vi "Main_24a.vi"() -> ()   [LabVIEW 2023]
uses:
  RB ENUM_Position ID.ctl
  Cluster _Point Location.ctl
  0c90424e-a446-4045-a5ae-fd3bd7481f50.vi
  <vilib>/Comparison/Equal/Equal Functor/Equal Functor.lvclass
panel:
  in  "Description":string="--- Day 24: Blizzard Basin ---\nWith everything replanted for next year (and with elephants and monkeys to tend the grove), you and the Elves leave for the extraction point.\n\nPartway up the mountain that shields the grove is a flat, open area that serves as the extraction point. It's a bit of a climb, but nothing the expedition can't handle.\n\nAt least, that would normally be true; now that the mountain is covered in snow, things have become more difficult than the Elves are used to.\n\nAs the expedition reaches a valley that must be traversed to reach the extraction site, you find that strong, turbulent winds are pushing small blizzards of snow and sharp ice around the valley. It's a good thing everyone packed warm clothes! To make it across safely, you'll need to find a way to avoid them.\n\nFortunately, it's easy to see all of this from the entrance to the valley, so you make a map of the valley and the blizzards (your puzzle input). For example:\n\n#.#####\n#.....#\n#>....#\n#.....#\n#...v.#\n#.....#\n#####.#\nThe walls of the valley are drawn as #; everything else is ground. Clear ground - where there is currently no blizzard - is drawn as .. Otherwise, blizzards are drawn with an arrow indicating their direction of motion: up (^), down (v), left (<), or right (>).\n\nThe above map includes two blizzards, one moving right (>) and one moving down (v). In one minute, each blizzard moves one position in the direction it is pointing:\n\n#.#####\n#.....#\n#.>...#\n#.....#\n#.....#\n#...v.#\n#####.#\nDue to conservation of blizzard energy, as a blizzard reaches the wall of the valley, a new blizzard forms on the opposite side of the valley moving in the same direction. After another minute, the bottom downward-moving blizzard has been replaced with a new downward-moving blizzard at the top of the valley instead:\n\n#.#####\n#...v.#\n#..>..#\n#.....#\n#.....#\n#.....#\n#####.#\nBecause blizzards are made of tiny snowflakes, they pass right through each other. After another minute, both blizzards temporarily occupy the same position, marked 2:\n\n#.#####\n#.....#\n#...2.#\n#.....#\n#.....#\n#.....#\n#####.#\nAfter another minute, the situation resolves itself, giving each blizzard back its personal space:\n\n#.#####\n#.....#\n#....>#\n#...v.#\n#.....#\n#.....#\n#####.#\nFinally, after yet another minute, the rightward-facing blizzard on the right is replaced with a new one on the left facing the same direction:\n\n#.#####\n#.....#\n#>....#\n#.....#\n#...v.#\n#.....#\n#####.#\nThis process repeats at least as long as you are observing it, but probably forever.\n\nHere is a more complex example:\n\n#.######\n#>>.<^<#\n#.<..<<#\n#>v.><>#\n#<^v^^>#\n######.#\nYour expedition begins in the only non-wall position in the top row and needs to reach the only non-wall position in the bottom row. On each minute, you can move up, down, left, or right, or you can wait in place. You and the blizzards act simultaneously, and you cannot share a position with a blizzard.\n\nIn the above example, the fastest way to reach your goal requires 18 steps. Drawing the position of the expedition as E, one way to achieve this is:\n\nInitial state:\n#E######\n#>>.<^<#\n#.<..<<#\n#>v.><>#\n#<^v^^>#\n######.#\n\nMinute 1, move down:\n#.######\n#E>3.<.#\n#<..<<.#\n#>2.22.#\n#>v..^<#\n######.#\n\nMinute 2, move down:\n#.######\n#.2>2..#\n#E^22^<#\n#.>2.^>#\n#.>..<.#\n######.#\n\nMinute 3, wait:\n#.######\n#<^<22.#\n#E2<.2.#\n#><2>..#\n#..><..#\n######.#\n\nMinute 4, move up:\n#.######\n#E<..22#\n#<<.<..#\n#<2.>>.#\n#.^22^.#\n######.#\n\nMinute 5, move right:\n#.######\n#2Ev.<>#\n#<.<..<#\n#.^>^22#\n#.2..2.#\n######.#\n\nMinute 6, move right:\n#.######\n#>2E<.<#\n#.2v^2<#\n#>..>2>#\n#<....>#\n######.#\n\nMinute 7, move down:\n#.######\n#.22^2.#\n#<vE<2.#\n#>>v<>.#\n#>....<#\n######.#\n\nMinute 8, move left:\n#.######\n#.<>2^.#\n#.E<<.<#\n#.22..>#\n#.2v^2.#\n######.#\n\nMinute 9, move up:\n#.######\n#<E2>>.#\n#.<<.<.#\n#>2>2^.#\n#.v><^.#\n######.#\n\nMinute 10, move right:\n#.######\n#.2E.>2#\n#<2v2^.#\n#<>.>2.#\n#..<>..#\n######.#\n\nMinute 11, wait:\n#.######\n#2^E^2>#\n#<v<.^<#\n#..2.>2#\n#.<..>.#\n######.#\n\nMinute 12, move down:\n#.######\n#>>.<^<#\n#.<E.<<#\n#>v.><>#\n#<^v^^>#\n######.#\n\nMinute 13, move down:\n#.######\n#.>3.<.#\n#<..<<.#\n#>2E22.#\n#>v..^<#\n######.#\n\nMinute 14, move right:\n#.######\n#.2>2..#\n#.^22^<#\n#.>2E^>#\n#.>..<.#\n######.#\n\nMinute 15, move right:\n#.######\n#<^<22.#\n#.2<.2.#\n#><2>E.#\n#..><..#\n######.#\n\nMinute 16, move right:\n#.######\n#.<..22#\n#<<.<..#\n#<2.>>E#\n#.^22^.#\n######.#\n\nMinute 17, move down:\n#.######\n#2.v.<>#\n#<.<..<#\n#.^>^22#\n#.2..2E#\n######.#\n\nMinute 18, move down:\n#.######\n#>2.<.<#\n#.2v^2<#\n#>..>2>#\n#<....>#\n######E#\nWhat is the fewest number of minutes required to avoid the blizzards and reach the goal?"
  out "Array":T1[][](array[typedef])
  in  "Example 2":string="#.######\n#>>.<^<#\n#.<..<<#\n#>v.><>#\n#<^v^^>#\n######.#"
  out "Answer":i32
  in  "Puzzle":string="#.######################################################################################################################################################\n#>v<<.^vvv^vv.^^>>v<>><v^<<.>^>v>v<v^vvvvvv^><^<vv<^^^v<vv>vvv.^v>.<>>v^v><<>^<<^vv<<>><<v<v<^v<..^>>vv^><<<v<^^><<<>>>vvv^.^.v>.^v^^.vv>^vv^>^^^><v<<<#\n#.<<v^><<.<>>>>^.<^<^^<>>^.^^.^v<vvv>>vv<^>.>>^^<<<^^>><^><<<v^>v.^^<.<<^v^>^^>.^.v^>.><<vv^>><>^....^<vv^><<^>v<v<^vvv<v<<><^vv<^>v^^^^^^^.^vv<^^<vvv<#\n#<>.v^.v<^><><v^^>>^><.v>^v^vv><><>>^>^v<^>>v^>^vvv^v..>vv>.^vv^<^.<.<v>>^<><v>^>^v..^>^><>vvv<v>^.>>^^<v^v>^<^vv.>.^v><v>v^>.^v<v>.<<vvv><^v^<^<^<vv<>#\n#>v..v^<^^v<><^^>vv>v^^^<^.^<<><^^^v>^<^v<<^>^<<.^><<^>>v^.v.><>>^<<><^^>>v>.^<^<vv><<>..>>v^^^>v>^<vv>.^>^<.^^v<>v>^.^>^^>.^v^>>^v>>>^<<^.^>><>v^>v>v.#\n#>^^^^^v^>>>^^v^v^v>v^v<v^.><<.^..v<^<^<^><<><<<>>v<<>><<^v^^>v>v<>.<vv>^<<<><.v<v<>>v^v<>>^v><.v>><<v><v<vv<<^^<><.^>v>^<^<^>^^.<.v>v^>>>><<<^v.vv<.<>#\n#>vv<vv^v<.<<v><<<^v>v<><vv<<vv<<.^.v>>v>.>v<^<<>v>>vv>..>v<^.v<.^<.>.<<<>>>^v>.^>>>>><<<^>..>>>^<^<>^>><>^><><v>v<<<v^.vvvv<v>>vv^>>>^.v^<>^><.<v>>v>>#\n#>>v.>><v^>v^v.<^.<vvv<<<v<>.^^v<<^^>>^^v^^.^.<>^vv^>>v<>^>v^.vv^v>.v^<>>v<<v<^>^vv^^v^><>v>.^<v<v<.^>>vvv>v^<^vv^<v^<<>^<v<>v<<v<<>v^v><>^vv^<<<^v>^>>#\n#<^<^>><<.<<.><<v>vv>v^v<<>..v<^>v^<.vv><v^<<<.v>v>>><<^.<v^vvv^<^v<<^^^^<v<<.<<^><v.<>>^><v>..<><vvv<.<>><.v>.v><<>vv<>.<<v.>><>>v<v^>^>>..>.<<^>^>^.>#\n#<v.>v>v<>>v^v>^v<^vv>^^>^vv>v<^^vv><^.<v<^<v>^>^v<v.<^<>^>>>vvvv<v>>^^<v.^v<^^<.<<<><v^<>^^<vvv><<>...^<><>^>vvv^^v..v..v^><^<>^>vv><v<^^vv^vvv>v^<v><#\n#<^^^^.>v>><<>v<vv<^<<^>v..vv^vvv>>>v<<^vv^^><^>^>^v.<<^v^^><vv>.>v..v.^v><^<^>>^>vv<<v.v>.<.>^.>>>^>>^^v^>^<.<><v>v^.^..<>.>^<^^<v.^v>^^^<<^v>>.>vv<v>#\n#>^^v>v.<v<<v..>><>..^v><>.^<v.>vv<>v^^>v.^v<<<vv>>v.^>><<^<v><v^.>>>^v>^>>v<<...<^^^vv.v^><<<>^^v<v^>v<v>.vv^vv.>>v<>><>v><vv>^>>v^..vv>v>^^>vvv>.>^v<#\n#<v>^^.<.^vv^<>^vv<<<<<vv^<^^<>v>^vv<>v<<>vv^<<v><<.^^..>.^>vv<^<>>^.<<<<<>.v>v><>.>v>v^<>^>vvv>.<^v^.>^<<v<^vvv^>v><<v^>.^><^><>v.^^<><vv<>.v..^<<v^>>#\n#<>^.>.><><v^<v>v>^<<>^v..<.<><>>^.vv>v.vv.>><>v^>.^><.<v.>v..^^v.^v^>^<^^<>>>v<^>>v<^<v^^^v<^v.vv<v^.><^^v^>^^^<.>.<v<.<v>^.><^^<v^<<^^v<.>>v>.vvv>v>>#\n#<v><v.^^<>v>.>^^^^>v<<v..v>><>v^.>^^<^>v<>v^v<v^<><^<>v>v^.<.^v^<^<>v^^<<^v><^.>^.v><><>>^v^v><.>v><<>v>v^.vvv><>^>>v^<<^v>^vv><><.^^>>vv^^v><^..>^v<>#\n#>v><^<vv^v>v><>v^<<><<^>v^v<^<^<v>><v^vv<<.vv<^v.><<<v.v.^<v<v.^^>><>^vv>v<v^>v^.<<><^<<.<vv<^.^>^^vv<^vv^..<^>^^<^^vvvv<><^^^<v<vv<v^>^v<^v><^^<..<v>#\n#>v^<<><<<^v.vvv>v<<v>>.^>^<^><..>>>^v.v.<<v<>>^^..><<v>vv^^<v<<^<>^v<^<<^.v>^<^>vv.>>>^>^^.<^<v<<^^v^^<><.>^.<><vv^<^>^>>^^vv^<^^^<^>^.v^<.<^^<.>v>v>>#\n#>^<v>v^<^>>..v<.><<<^><^v>vv<>^^v<v^vv><<<><^v<^.v<^>v<v<^<v>v>^v^^>>^<<^.<<v<vvv><^>v>^<>v>v^^>.<vv<<>>^^<>vv>^v^.><^^^vv>v<<<<v^v<vv><.<v<^v>>^v>v<>#\n#<vv^>^^<v>^v>>.^.<<^<^^.v>>vv>^<><><>>^>>>vv<.v<^<<<vvv.>v<>>^>>v<>>..>^v^>^>^v<<>v^v^.^>^v^^v>.><v<<.v<v>vv>>.<<v.v.^<>><>vv>^^>><^^.<>>>vv<<>^>><<<.#\n#<^<^^.>>>^<>^v<^v<<>v^<>^vv<^^v<v<<^^.><<vv>v^<^^<>^^^v<v>^.^^<<^v<v^.^>>>><v>><>>>><v<^^<v>v^v>^>v>v^^^<>v><v><.>><>^vvvvv>vv<<v^^<v^v>v.^v<vv<^.^^v<#\n#..>^>>^^^^v<>>^><^^v>^^>v.><>><vv<><^.<><^v.^vv<><v>v^<<v>v<vv<><>v^.^<<<vv>>^^<<>^.v<^.v^^<>>>^v<.>^..^^^<<<>..v<><v<>v<>>..<v><>^^>>.<>v<<>v>.<v^vv.#\n######################################################################################################################################################.#"
  in  "Example":string="#.#####\n#.....#\n#>....#\n#.....#\n#...v.#\n#.....#\n#####.#"
  # "326"
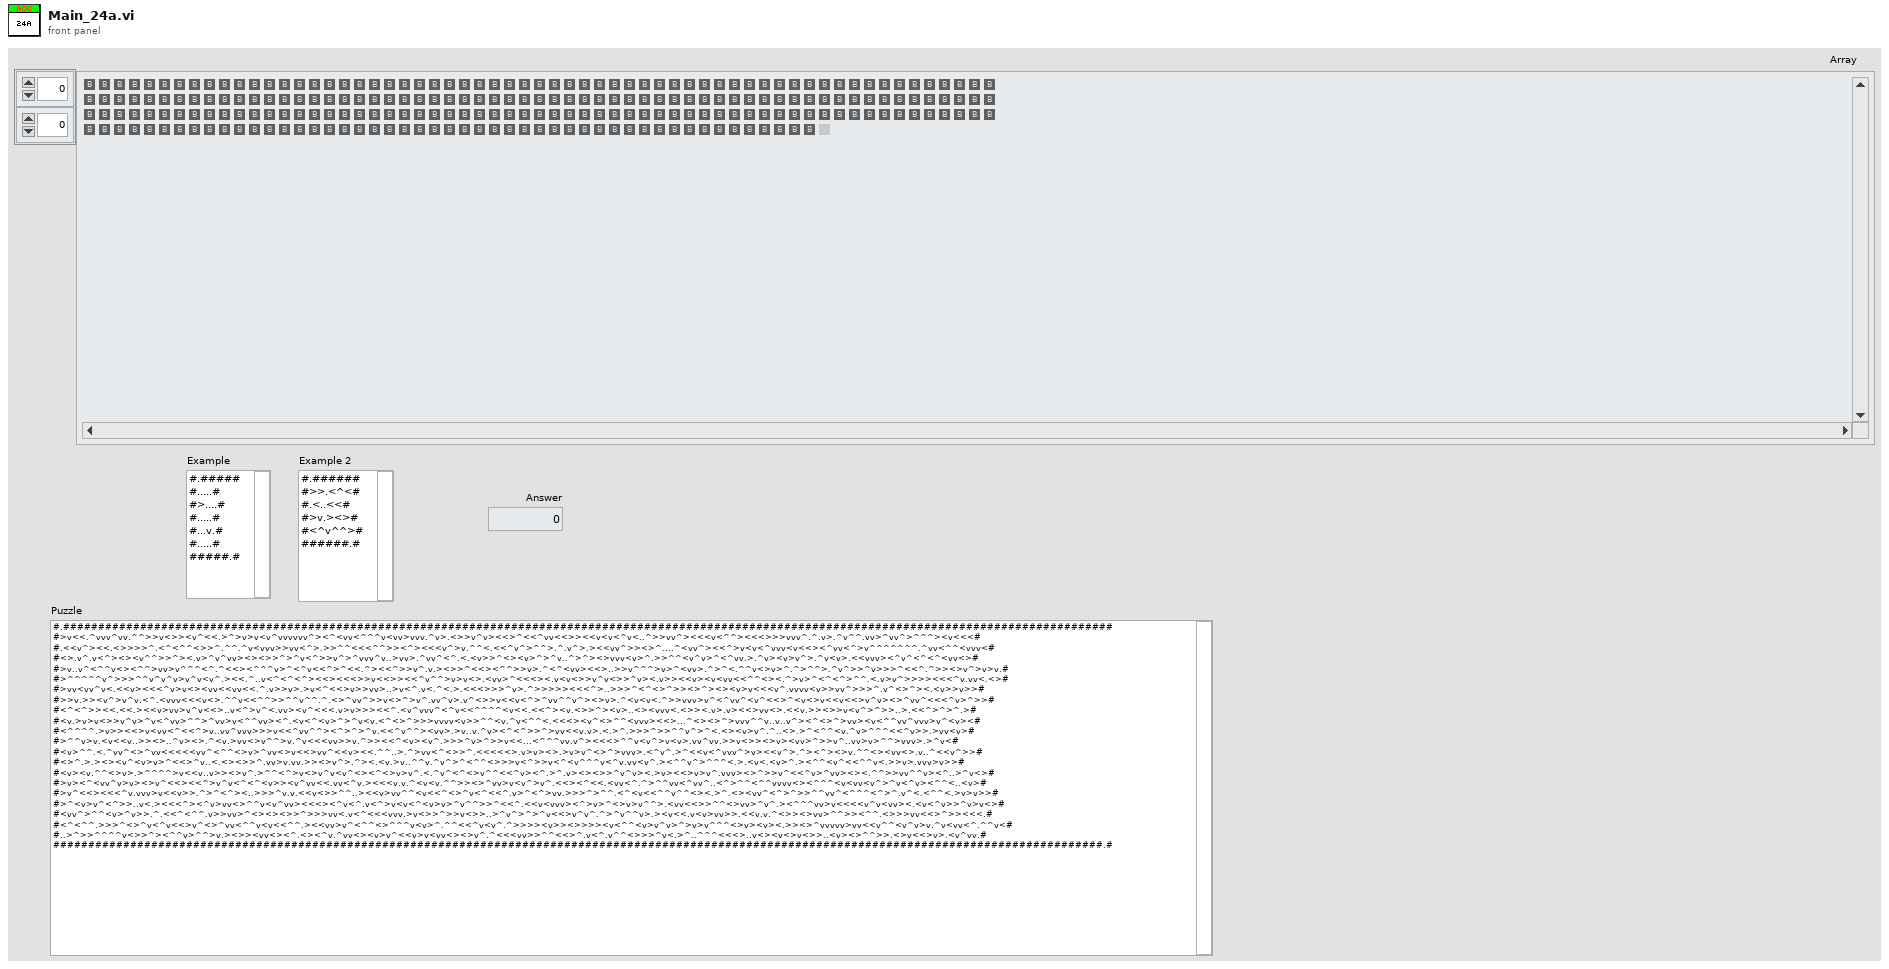
[diagram p1: front panel]
types:
  T1 = typedef "RB ENUM_Position ID.ctl" = enum32{"Blank", "Wall", "UP", "Down", "Left", "Right", "Two", "Three", "Four", "Spot"}
  T2 = typedef "Cluster _Point Location.ctl" = cluster{"X col":i32, "Y row":i32}
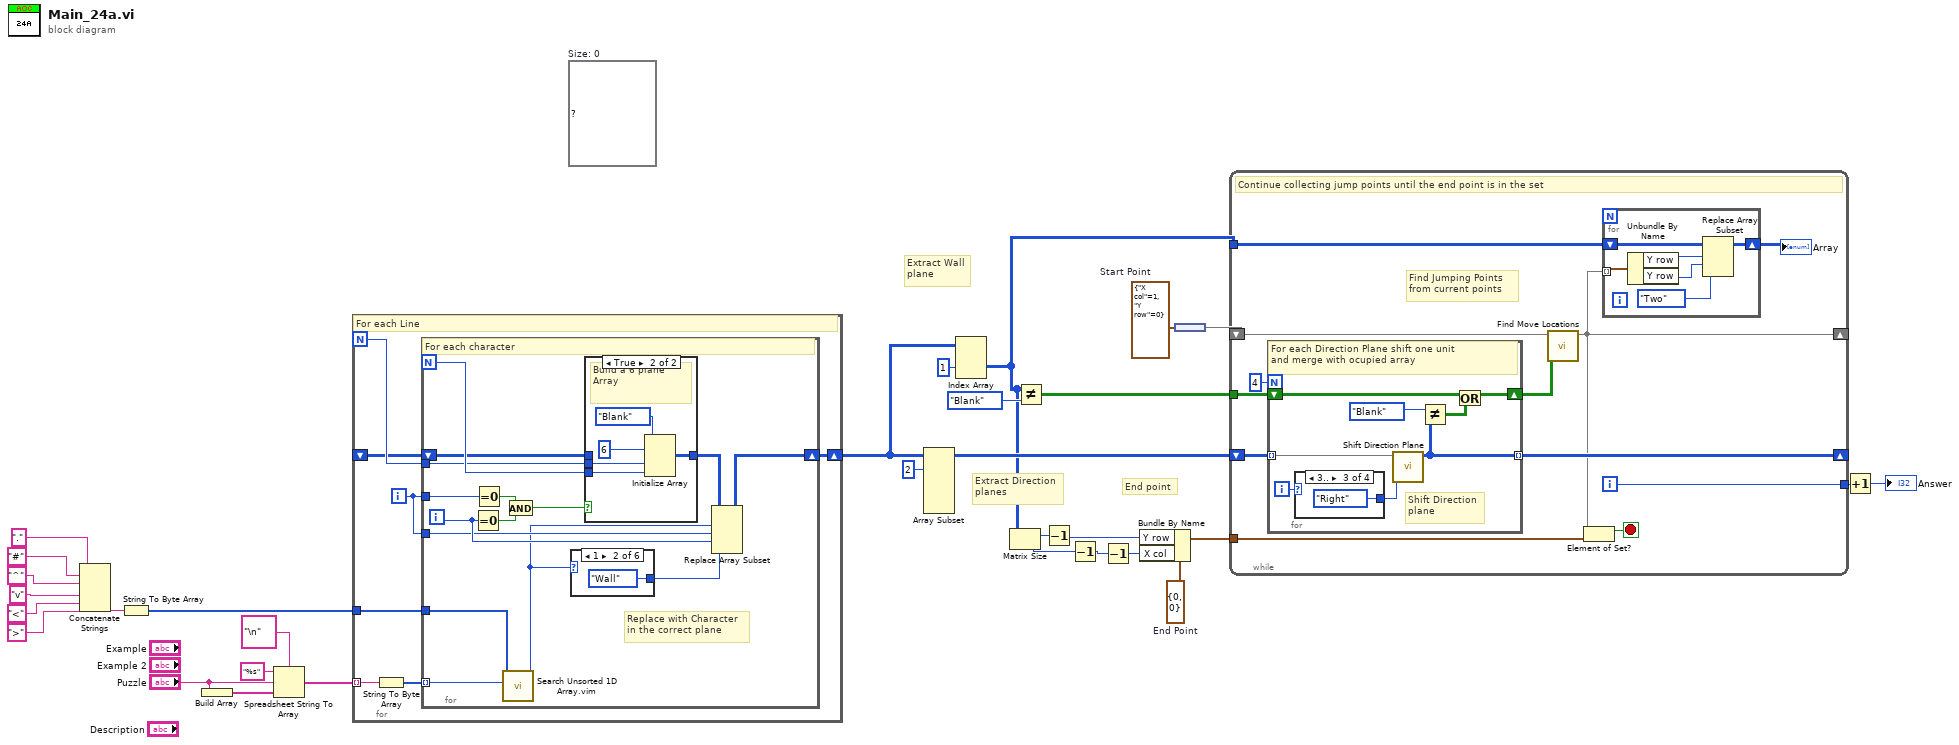
[diagram p0: block diagram]
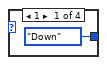
[diagram p2: hidden frame]
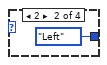
[diagram p3: hidden frame]
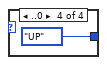
[diagram p4: hidden frame]
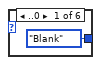
[diagram p5: hidden frame]
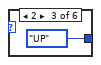
[diagram p6: hidden frame]
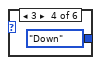
[diagram p7: hidden frame]
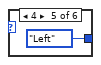
[diagram p8: hidden frame]
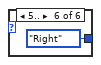
[diagram p9: hidden frame]
diagram:
  w13 = T2 {"X col"=0, "Y row"=0}  # End Point
  w5 = T2 {"X col"=1, "Y row"=0}  # Start Point
  (unwired) map{T2, u32} {}  # Size: 0
  # "End point"
  # "Extract Wall\nplane"
  # "Extract Direction\nplanes"
  n1 = Concatenate Strings(".", "#", "^", "v", "<", ">") -> (w23:string)
  n2 = String To Byte Array(string=w23) -> (unsigned byte array=w22:u8[])
  n3 = Build Array("Puzzle") -> (w31:string[])
  n4 = Spreadsheet String To Array(delimiter (Tab)="\n", format string="%s", spreadsheet string="Puzzle", array type (2D Dbl)=w31) -> (array=w28:string[])
  n5 = for {
    N -> [w36]
    tunnel: w28 -> [w38] mode=indexing
    shift-right: [w35] -> w16
    shift-left: _ -> [w34]
    tunnel: w22 -> [w33]
    i -> [w32]
    # "For each Line"
    n6 = String To Byte Array(string=w38) -> (unsigned byte array=w37:u8[])
    n7 = for {
      N -> [w49]
      tunnel: w37 -> [w44] mode=indexing
      tunnel: w32 -> [w53]
      tunnel: w36 -> [w48]
      shift-right: [w39] -> w35
      shift-left: w34 -> [w47]
      tunnel: w33 -> [w46]
      tunnel: w32 -> [w42]
      i -> [w43]
      # "Replace with Character\nin the correct plane"
      # "For each character"
      n8 = Equal To 0?(x=w43) -> (x = 0?=w51:bool)
      n9 = Equal To 0?(x=w53) -> (x = 0?=w52:bool)
      n10 = call "Search Unsorted 1D Array.vim"("element"=w44, "unsorted 1D array"=w46) -> ("index of element"=w41:i32)  [unwired: 9 in]
      n11 = And(x=w52, y=w51) -> (x .and. y?=w50:bool)
      n12 = case shown="1" w41 {
        tunnel: [RB_ENUM_Position_ID."Blank" ("Position") RB_ENUM_Position_ID."Wall" ("Position") RB_ENUM_Position_ID."UP" ("Position") RB_ENUM_Position_ID."Down" ("Position") RB_ENUM_Position_ID."Left" ("Position") RB_ENUM_Position_ID."Right" ("Position")] -> w40
        frame ..0 {
        }
        frame 1 {
        }
        frame 2 {
        }
        frame 3 {
        }
        frame 4 {
        }
        frame 5.. {
        }
      }
      n13 = case shown="True" w50 {
        tunnel: w49 -> [_ w62]
        tunnel: w48 -> [_ w63]
        tunnel: [w60 w64] -> w45
        tunnel: w47 -> [w60 _]
        frame False {
        }
        frame True {
          # "Build a 6 plane\nArray"
          n14 = Initialize Array(RB_ENUM_Position_ID."Blank" ("Position"), 6 ("dimension size"), w63, w62) -> (w64:T1[][][])
        }
      }
      n15 = Replace Array Subset(array=w45, new element=w40, index (dim 0)=w41, index (dim 1)=w42, index (dim 2)=w43) -> (w39:T1[][][])
    }
  }
  n16 = Array Subset(array=w16, index (dim 0)=2 ("index")) -> (w15:T1[][][])  [unwired: 5 in]
  n17 = Index Array(array=w16, index (dim 0)=1 ("index (page)")) -> (element=w2:T1[][])  [unwired: 2 in]
  n18 = Matrix Size(0:w2) -> (1:w14:i32, 2:w10:i32)
  n19 = Not Equal?(x=w2, y=RB_ENUM_Position_ID."Blank" ("Position")) -> (x != y?=w12:bool[][])
  n20 = Decrement(x=w14) -> (x-1=w8:i32)
  n21 = Decrement(x=w10) -> (x-1=w11:i32)
  n22 = Decrement(x=w11) -> (x-1=w9:i32)
  n23 = Bundle By Name(cluster=w13, "Y row"=w8, "X col"=w9) -> (w7:T2)
  n24 = node(w5) -> (w4:set{T2})
  n25 = while {
    shift-right: [w74] -> _
    shift-left: w15 -> [w77]
    shift-right: [w67] -> _
    shift-left: w4 -> [w70]
    tunnel: w12 -> [w75]
    tunnel: w7 -> [w72]
    tunnel: [w71] -> w6
    tunnel: w2 -> [w68]
    i -> [w71]
    stop <- w73 stop-if-true
    # "Find Jumping Points\nfrom current points"
    # "Continue collecting jump points until the end point is in the set"
    n26 = for {
      N: 4 -> [_]
      shift-right: [w86] -> w69
      shift-left: w75 -> [w87]
      tunnel: w77 -> [w84] mode=indexing
      tunnel: [w85] -> w74 mode=indexing
      i -> [w91]
      # "Shift Direction\nplane"
      # "For each Direction Plane shift one unit\nand merge with ocupied array"
      n27 = case shown="3.." w91 {
        tunnel: [RB_ENUM_Position_ID."Down" ("Position") RB_ENUM_Position_ID."Left" ("Position") RB_ENUM_Position_ID."Right" ("Position") RB_ENUM_Position_ID."UP" ("Position")] -> w90
        frame 1 {
        }
        frame 2 {
        }
        frame 3.. {
        }
        frame ..0 {
        }
      }
      n28 = call "Shift Direction Plane.vi"("Direction"=w90, "Direction Plane"=w84) -> ("Direction Plane Out"=w85:T1[][])  [unwired: 9 in]
      n29 = Not Equal?(x=RB_ENUM_Position_ID."Blank" ("Position"), y=w85) -> (x != y?=w88:bool[][])
      n30 = Or(x=w87, y=w88) -> (x .or. y?=w86:bool[][])
    }
    n31 = call "Find Move Locations.vi"("Ocupied array"=w69, "Jump Points"=w70) -> ("Jump Points"=w67:set{T2})  [unwired: 9 in]
    n32 = Element of Set?(10:w72, 11:w67) -> (3:w73:bool)
    n33 = for {
      shift-right: [w82] -> w66
      shift-left: w68 -> [w83]
      tunnel: w67 -> [w81] mode=indexing
      n34 = Unbundle By Name(w81) -> ("Y row"=w80:i32, "Y row"=w79:i32)
      n35 = Replace Array Subset(array=w83, new element=RB_ENUM_Position_ID."Two" ("Position"), index (row)=w80, index (col)=w79) -> (w82:T1[][])
    }
    "Array" <- w66
  }
  n36 = Increment(x=w6) -> (x+1=→"Answer":i32)
